vi "Dashboard Main.vi"() -> ()   [LabVIEW 2018]
uses:
  <vilib>/Utility/miscctls.llb/LVRowAndColumnTypeDef.ctl
  <vilib>/event_ctls.llb/eventvkey.ctl
  <vilib>/Rock Robotics/WPI/Dashboard/WPI_DashboardLogging Global.vi
  Personalities Tool/Main.vi
  <vilib>/Rock Robotics/Network Tables/NT Read Boolean.vi
  <vilib>/FTP/NI_FTP.lvlib
  Personalities Tool/Personalities Tool.lvlib
panel:
  in  "Camera Settings Right":T1={"Frame Rate"=30, "Compression"=30, "Size"=1, "DB Camera Config"=FALSE} {"Frame Rate" scale=1.0..30.0; "Compression" scale=100.0..-1.0; "Size" items=["640x480", "320x240", "160x120"]}
  in  "Camera Name Right":string(combo)="No Camera Selection"
  out "Camera Perf":string
  in  "Camera Settings":T1={"Frame Rate"=30, "Compression"=30, "Size"=1, "DB Camera Config"=FALSE} {"Frame Rate" scale=1.0..30.0; "Compression" scale=100.0..-1.0; "Size" items=["640x480", "320x240", "160x120"]}
  in  "TCP":refnum<k5>
  in  "Rec Mode":enum32{"Stop", "Record", "Playback"}(radio)
  out "Robot IP":string
  out "Image Message":string="Timeout in Camera Communications"
  in  "Dashboard Tab":T2(tab)
  out "Personality":string
  out "Elevator State":string
  out "Elevator Position":string
  in  "Select Auto":string(combo)="Select Autonomous ..."
  out "NT Connection":bool
  out "JS1 Z":dbl(slide) scale=-1.0..1.0 scale format="%#_2e"
  out "JS1 Graph":cluster{"X":dbl, "Y":dbl}[](graph)
  out "JS1 Buttons":T3
  out "JS2 Z":dbl(slide) scale=-1.0..1.0 scale format="%#_2e"
  out "JS2 Graph":cluster{"X":dbl, "Y":dbl}[](graph)
  out "JS2 Buttons":T3
  out "Mode":T4(ring)=enum."Auto Disabled"
  out "Right Camera Perf":cluster{"Bandwidth (Mbps)":dbl, "FPS":dbl}
  out "BirdBeak State":bool
  out "Camera Image Right":T5(plugin-control)
  in  "DB/String 9":string
  in  "DB/String 8":string
  in  "DB/String 7":string
  in  "DB/String 6":string
  in  "DB/String 5":string
  in  "DB/String 4":string
  in  "DB/String 3":string
  in  "DB/String 2":string
  in  "DB/String 1":string
  in  "DB/String 0":string
  in  "DB/Slider 0":dbl(slide) scale=0.0..5.0
  in  "DB/Slider 1":dbl(slide) scale=0.0..5.0
  in  "DB/Slider 2":dbl(slide) scale=0.0..5.0
  in  "DB/Slider 3":dbl(slide) scale=0.0..5.0
  out "DB/LED 3":bool
  out "DB/LED 2":bool
  out "DB/LED 1":bool
  out "DB/LED 0":bool
  in  "DB/Button 3":bool
  in  "DB/Button 2":bool
  in  "DB/Button 1":bool
  in  "DB/Button 0":bool caption="New Name"
  in  "Open Personalities Tool":bool
  in  "Retrieve File":bool
  in  "Click me if this is a new Driver Station":bool
  out "String":string
  out "Error":bool
  in  "Transfer File":bool
  in  "Edit File":bool
  in  "File":u16(ring) items=["CodeConstants.ini", "CodeConstants_Comp.ini", "CodeConstants_Prac.ini", "ConfigFileSettings.ini", "ElevatorBot.ini", "NewConfigFile.ini", "Outlaw.ini", "PacBot.ini"]
  in  "Test Slider":dbl(slide) scale=0.0..100.0 scale format="%#_3g"
  in  "On/Off":bool caption="Solenoid"
  in  "Test Name":u16(ring) items=["Select the test to run..."]
  in  "Test Tree":string(tree)
  in  "Motor":cluster{"Value":dbl, "Enable":bool} {"Value" scale=-1.0..1.0 scale format="%#_3g"}
  out "Progress":T6 {"Test Progress" scale=0.0..100.0}
  in  "Rev/Fwd":cluster{"Forward":bool, "Reverse":bool}
  in  "Test Ring":u16(ring) items=["Monochrome", "Color"]
  out "Cmd Status":string
  in  "Execute Command":bool
  in  "Command Params":string[][](table)
  in  "Command Selection":i32(listbox)
  in  "CheckList":i32(listbox)
  out "Tree":string(tree)
  out "Camera Image":T5(plugin-control)
  out "Background":bool
  in  "Camera Name":string(combo)="No Camera Selection"
  # "HW"
  # "HW"
  # "Joysticks"
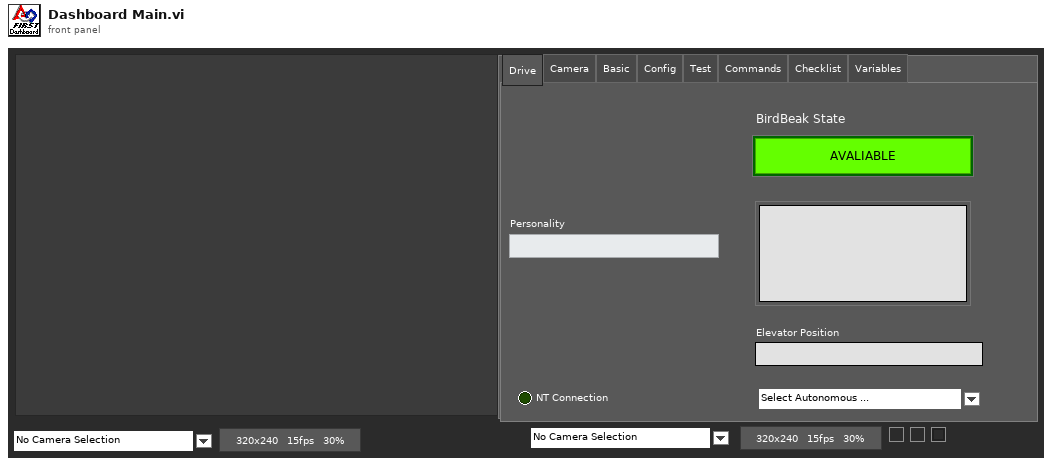
[diagram p1: front panel]
types:
  T1 = cluster{"Frame Rate":i32, "Compression":i32, "Size":u16, "DB Camera Config":bool}
  T2 = enum32{"Drive", "Camera", "Basic", "Config", "Test", "Commands", "Checklist", "Variables"}
  T3 = cluster{bool, bool, bool, bool, bool, bool, bool, bool, bool, bool, bool, bool}
  T4 = enum8{"Tele-Op Disabled", "Tele-Op Enabled", "Auto Disabled", "Auto Enabled", "Test Disabled", "Test Enabled", "Disconnected", "No Code", "E-Stop"}
  T5 = typedef "IMAQ Image.ctl" = refnum<image>
  T6 = cluster{"Test Progress":u8, "Test Progress Text":string}
  T7 = cluster{"Save Path":path, "Interval (s)":dbl, "Keep":i32}
  T8 = enum32{"Drive", "Camera", "Basic", "Custom", "Test", "Commands", "Checklist", "Variables"}
  T9 = typedef "Image Type" = u32
  T10 = cluster{"IDs":cluster{"RPC field ID":u16, "Unique ID":u16}, "String":string}
  T11 = cluster{"Error Strings":string, "Disable Counts":cluster{u16, u16}, "Rail Faults":cluster{u16, u16, u16}, "Robot IP":string, "DB Mode":u8, "Event Info":cluster{"Name":string, "Type":u8, "Number":u16, "Replay":u8}}
  T12 = cluster{"Storage":cluster{"Disk Free":u64, "RAM Block":u32, "RAM free":u32}, "CPU Utilization":cluster{"CPU % ISR":sgl, "CPU % Time Crit":sgl, "CPU % Timed Str":sgl, "CPU % High":sgl, "CPU % Above":sgl, "CPU % Normal":sgl, "CPU % Low":sgl}, "CAN":cluster{"% Bus Utilization":sgl, "Bus Off Cnt":u32, "TX_FIFO Full Cnt":u32, "Receive Error Cnt":u8, "Transmit Error Cnt":u8}, "HID":cluster{"HID Outputs":u32, "Rumble Low":u16, "Rumble High":u16}[]}
  T13 = cluster{"Status bits":cluster{"Test Mode":bool, "Autonomous":bool, "Enabled":bool, "Code Start":bool, "Brownout":bool, "Reserved 2":bool, "Reserved 3":bool, "E-Stop":bool}, "Code Trace":cluster{"Disabled":bool, "TeleOp":bool, "Auto":bool, "Test":bool}, "Controller Type":enum16{"unknown", "cRIO", "roboRio"}, "Code?":enum16{"unknown", "noCode", "code"}, "Battery V":dbl}
  T14 = cluster{"Control Bits":cluster{"TestMode":bool, "Autonomous":bool, "Enabled":bool, "FMS Present":bool, bool, bool, bool, "E-Stop":bool}, "Team Station ":u8, "Countdown":sgl, "Joystick Values":cluster{"Axes":dbl[], "Buttons":bool[], "POVs":i16[]}[]}
  T15 = cluster{"Axes":dbl[], "Buttons":bool[], "POVs":i16[]}[]
  T16 = cluster{"Axes":dbl[], "Buttons":bool[], "POVs":i16[]}
  T17 = cluster{"Buttons[0]":bool, "Buttons[1]":bool, "Buttons[2]":bool, "Buttons[3]":bool, "Buttons[4]":bool, "Buttons[5]":bool, "Buttons[6]":bool, "Buttons[7]":bool, "Buttons[8]":bool, "Buttons[9]":bool, "Buttons[10]":bool, "Buttons[11]":bool}
  T18 = cluster{"Camera Image":refnum<vi>, "Dashboard Tab":refnum<vi>, "Background":refnum<vi>, "Rec Mode":refnum<vi>, "Test Slider":refnum<vi>, "On/Off ":refnum<vi>, "Test Ring":refnum<vi>, "Rev/Fwd":refnum<vi>, "Test Name":refnum<vi>, "Motor":refnum<vi>, "Progress":refnum<vi>, "CheckList":refnum<vi>, "Tree":refnum<vi>, "Test Tree":refnum<vi>, "Command Params":refnum<vi>, "Command Selection":refnum<vi>, "Execute Command":refnum<vi>, "Cmd Status":refnum<vi>, "Camera Settings":refnum<vi>, "Camera Name":refnum<vi>, "Camera Perf":refnum<vi>, "Camera Settings Right":refnum<vi>, "Camera Name Right":refnum<vi>, "Camera Image Right":refnum<vi>}
  T19 = cluster{"Global Rectangle":i32[], "Contours":cluster{"Contour Type":u32, "ROI Type":u32, "Points":i32[]}[]}
  T20 = cluster{"Camera Name":string, string, "Saved DB Images Info":cluster{"Save Path":path, "Interval (s)":dbl, "Keep":i32}}
  T21 = cluster{"Camera Name Right":string, string, "Saved DB Images Info":cluster{"Save Path":path, "Interval (s)":dbl, "Keep":i32}}
  T22 = cluster{"Operation":enum16{"Update", "Clear"}, "Color Box":u32}[]
  T23 = enum32{"Invalid", "Standard", "Closed", "Hidden", "Minimized", "Maximized"}
  T24 = typedef "eventvkey.ctl" = enum16{"ASCII", "Enter", "Return", "Shift", "Ctrl", "Alt", "Cmd", "Opt", "Caps", "NumLock", "Clear", "Break", "Up", "Down", "Left", "Right", "Insert", "Delete", "Home", "End", "PageUp", "PageDown", "Escape", "Help", "Pause", "ScrollLock", "F1", "F2", "F3", "F4", "F5", "F6", "F7", "F8", "F9", "F10", "F11", "F12", "F13", "F14", "F15", "F16", "F17", "F18", "F19", "F20", "F21", "F22", "F23", "F24", "Play", "VolumeUp", "VolumeDown", "Mute", "Two Byte Char"}
  T25 = cluster{"Image Size":bool, "Image Type":bool, "Pixel Value":bool, "ROI Information":bool, "Zoom Factor":bool}
  T26 = cluster{"Operation":enum16{"Update", "Clear"}, "Color Box":u32}
  T27 = typedef "LVRowAndColumnTypeDef.ctl" = cluster{"Row":i32, "Column":i32}
  T28 = cluster{"Shift":bool, "Ctrl":bool, "Alt":bool, "Cmd":bool, "Opt":bool}
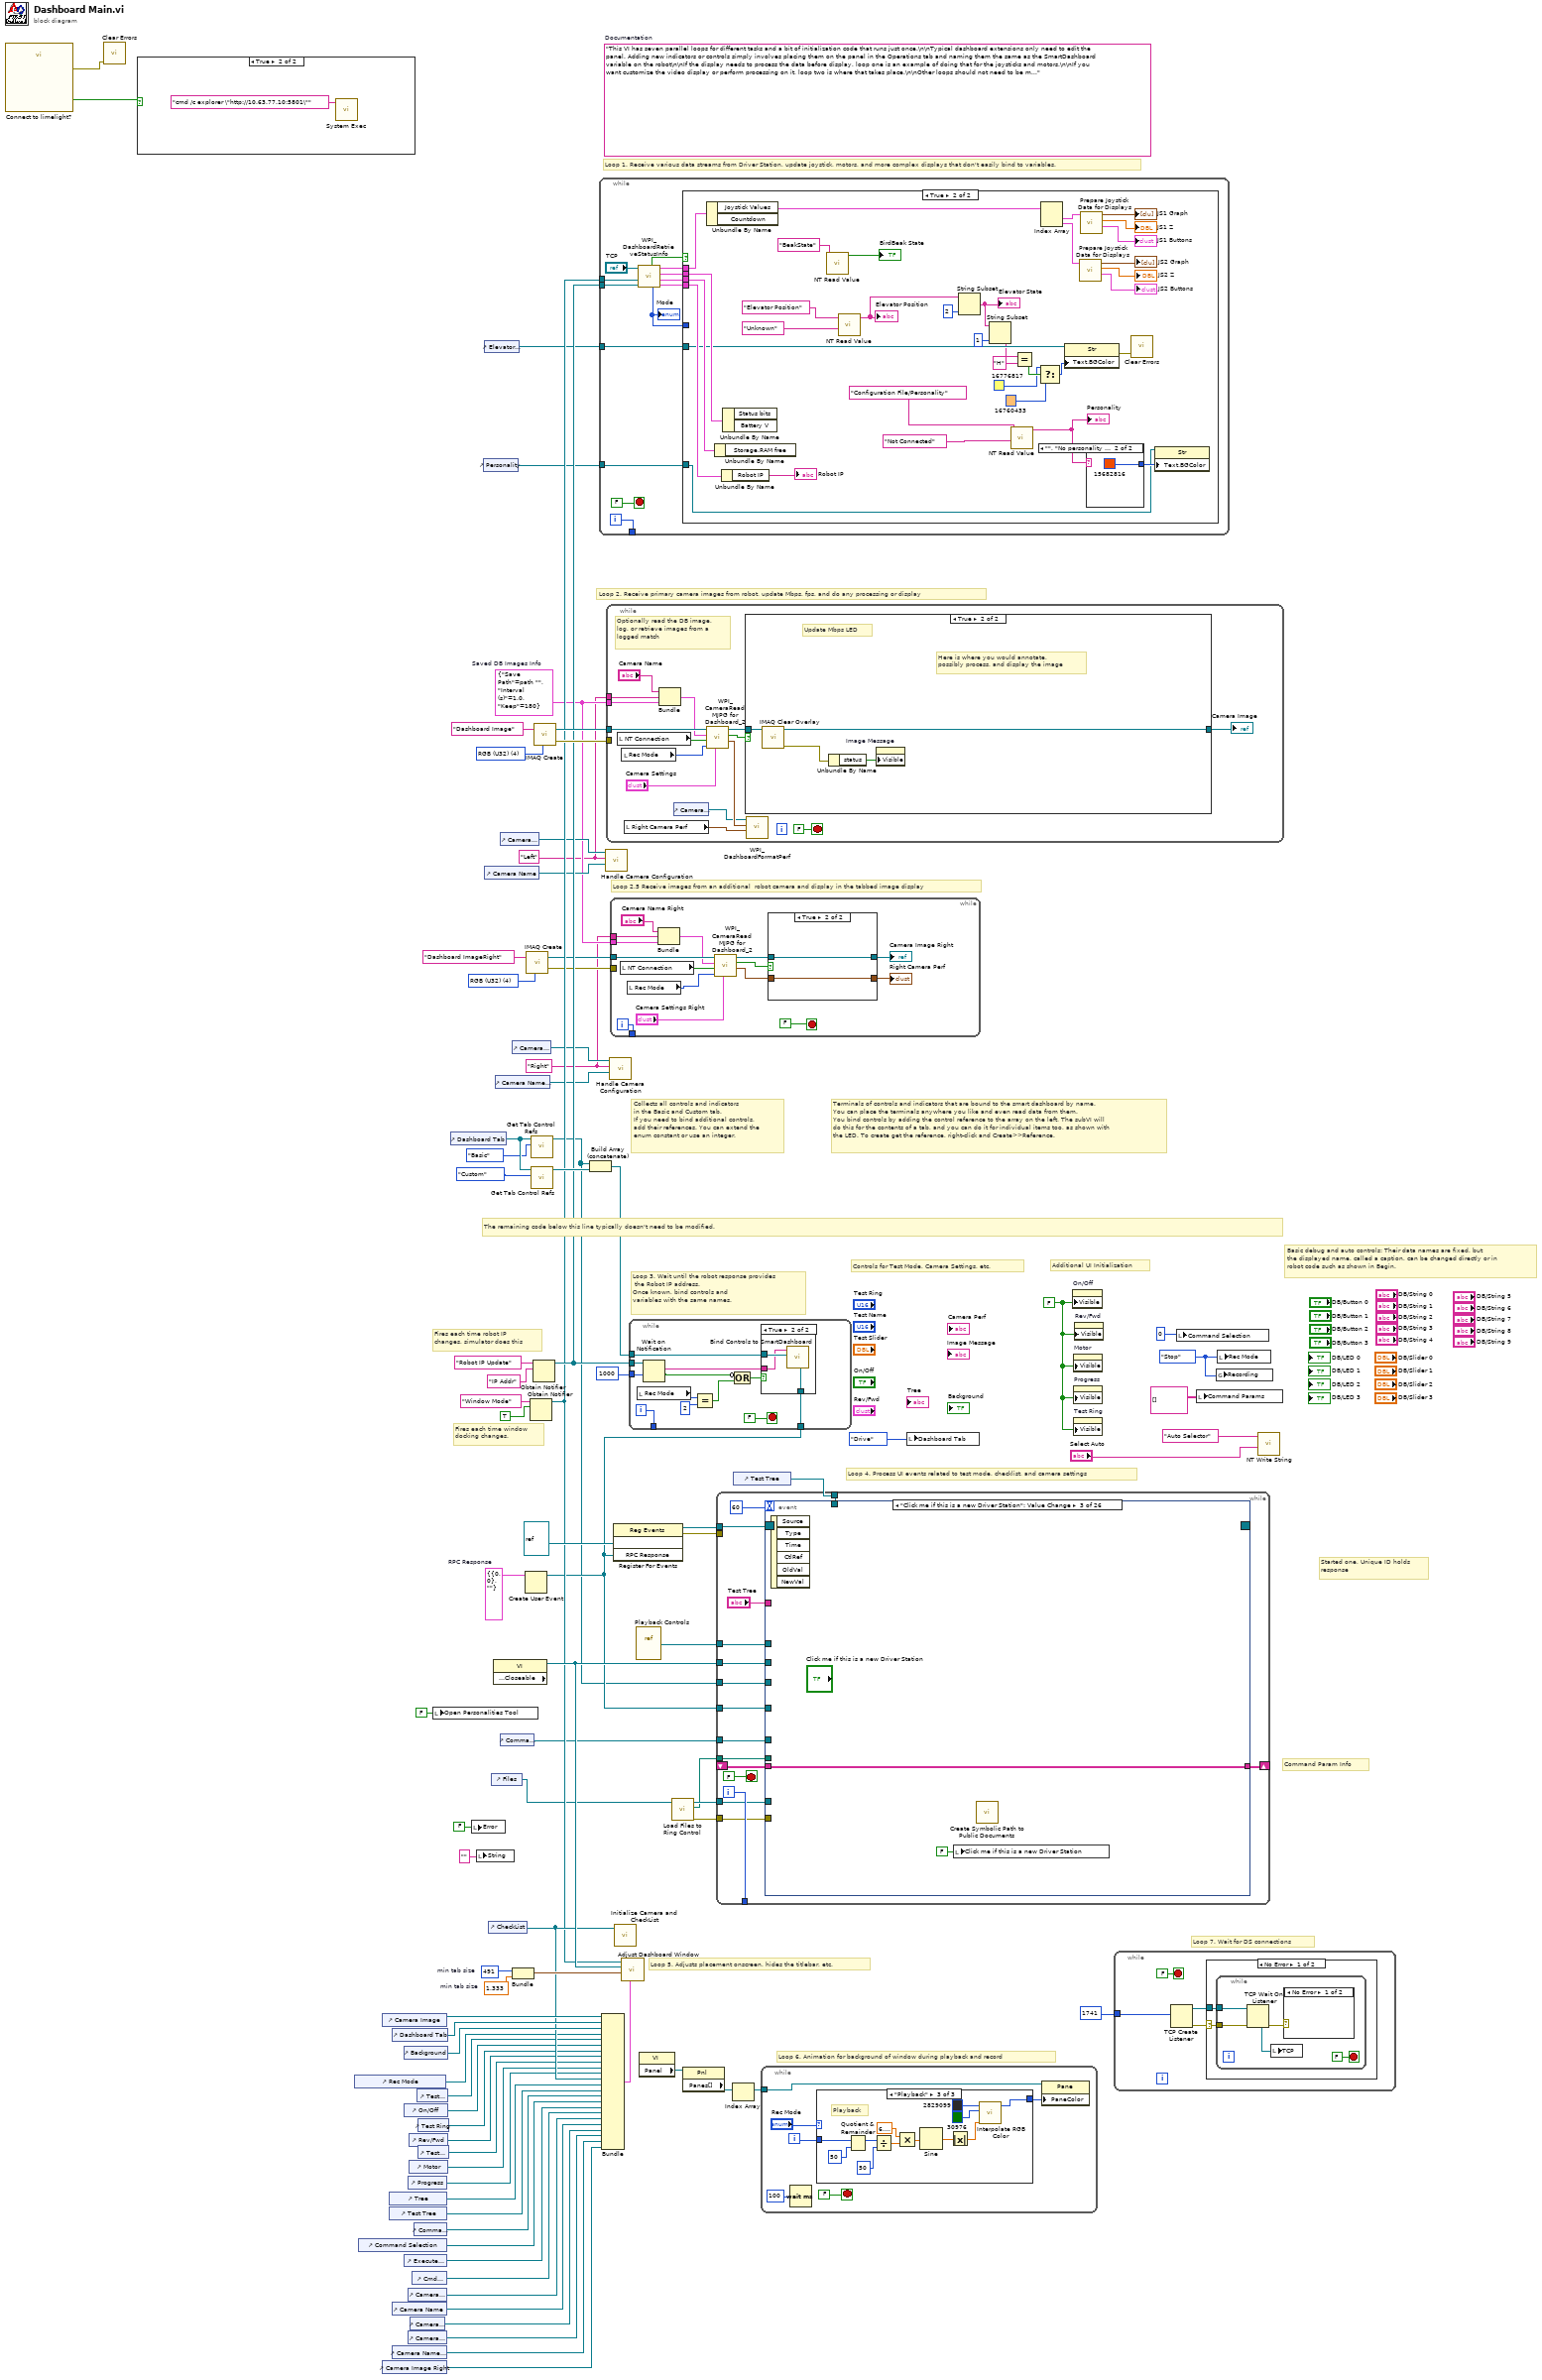
[diagram p0: block diagram]
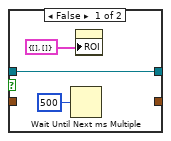
[diagram p3: hidden frame]
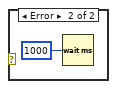
[diagram p4: hidden frame]
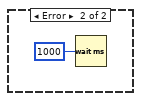
[diagram p5: hidden frame]
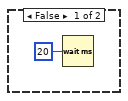
[diagram p6: hidden frame]
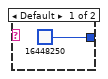
[diagram p7: hidden frame]
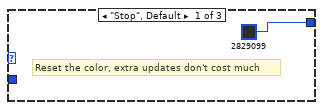
[diagram p8: hidden frame]
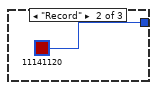
[diagram p9: hidden frame]
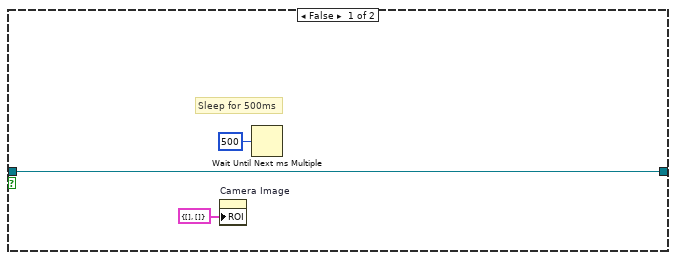
[diagram p11: hidden frame]
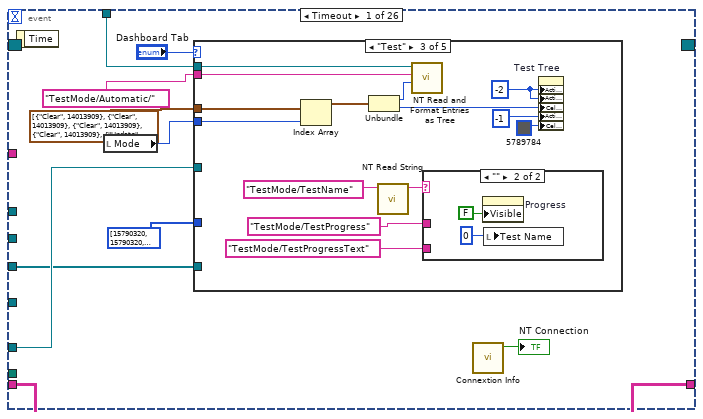
[diagram p12: hidden frame]
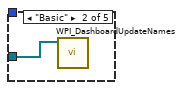
[diagram p14: hidden frame]
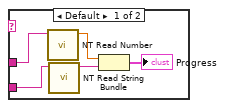
[diagram p15: hidden frame]
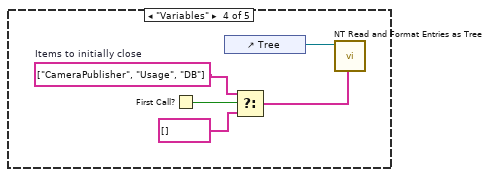
[diagram p16: hidden frame]
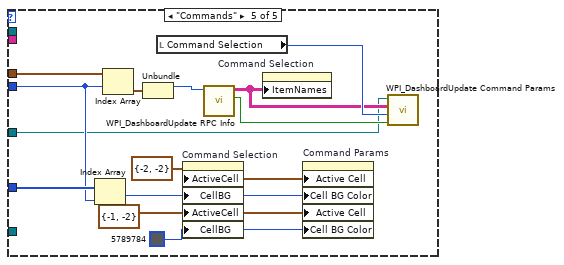
[diagram p17: hidden frame]
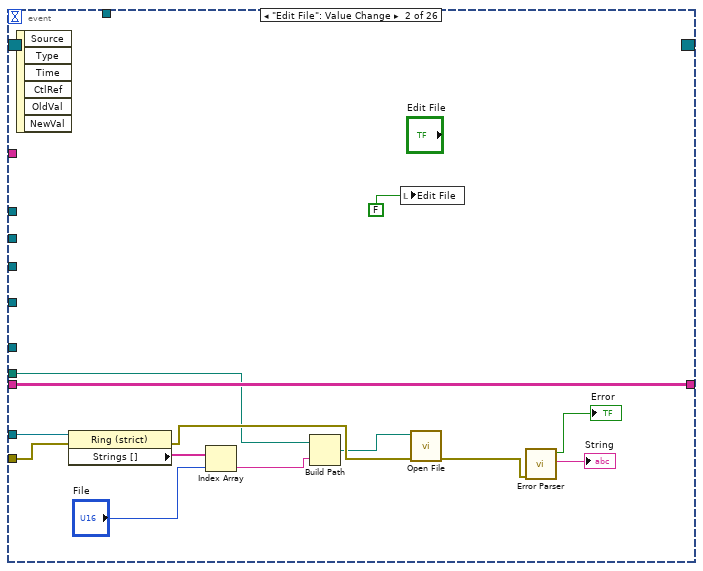
[diagram p18: hidden frame]
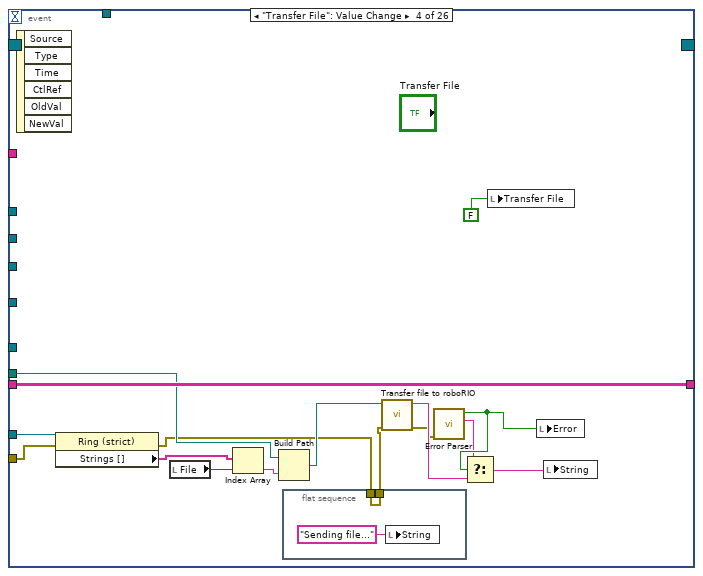
[diagram p19: hidden frame]
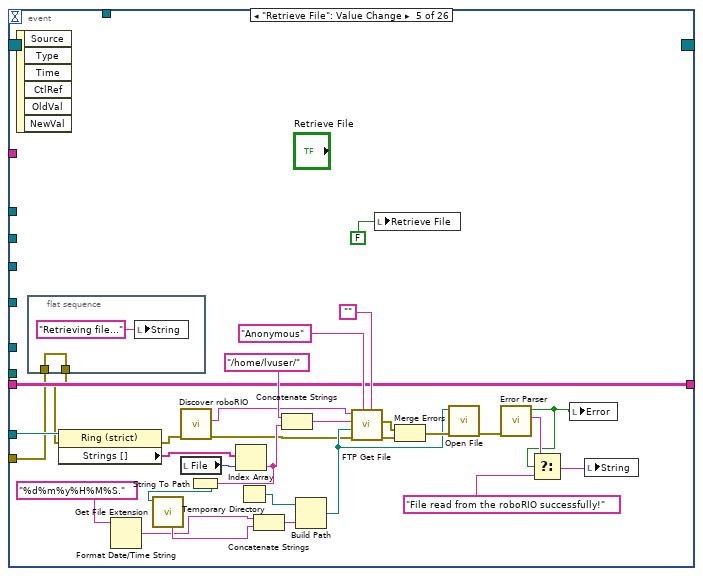
[diagram p20: hidden frame]
diagram:
  w14 = T7 {"Save Path"=path "", "Interval (s)"=1.0, "Keep"=180}  # Saved DB Images Info
  w13 = "Right"
  w12 = "Left"
  w24 = T9 4 items=["Grayscale (U8)", "Grayscale (I16)", "Grayscale (SGL)", "Complex (CSG)", "RGB (U32)", "HSL (U32)", "RGB (U64)"] ("Image Type")
  w40 = T10 {"IDs"={"RPC field ID"=0, "Unique ID"=0}, "String"=""}  # RPC Response
  w63 = 491  # min tab size
  w62 = 1.333  # min tab size
  w70 = enum32{"Stop", "Record", "Playback"}."Stop" ("Rec Mode")
  w47 = FALSE ("Visible")
  (unwired) "This VI has seven parallel loops for different tasks and a bit of initialization code that runs just once.\n\nTypical dashboard extensions only need to edit the panel. Adding new indicators or controls simply involves placing them on the panel in the Operations tab and naming them the same as the SmartDashboard variable on the robot\n\nIf the display needs to process the data before display, loop one is an example of doing that for the joysticks and motors.\n\nIf you want customize the video display or perform processing on it, loop two is where that takes place.\n\nOther loops should not need to be modified. They are pretty standard, and document the task they perform."  # Documentation
  w87 = T9 4 items=["Grayscale (U8)", "Grayscale (I16)", "Grayscale (SGL)", "Complex (CSG)", "RGB (U32)", "HSL (U32)", "RGB (U64)"] ("Image Type")
  # "Loop 2.5 Receive images from an additional  robot camera and display in the tabbed image display"
  # "Command Param Info"
  # "Started one, Unique ID holds\nresponse"
  # "Loop 7. Wait for DS connections"
  # "Basic debug and auto controls: Their data names are fixed, but\nthe displayed name, called a caption, can be changed directly or in\nrobot code such as shown in Begin."
  # "Controls for Test Mode, Camera Settings, etc."
  # "Additional UI Initialization"
  # "Loop 6. Animation for background of window during playback and record"
  # "Fires each time robot IP\nchanges, simulator does this"
  # "Fires each time window\ndocking changes."
  # "Collects all controls and indicators\nin the Basic and Custom tab.\nIf you need to bind additional controls,\nadd their references. You can extend the\nenum constant or use an integer."
  # "The remaining code below this line typically doesn't need to be modified."
  # "Loop 4. Process UI events related to test mode, checklist, and camera settings"
  # "Terminals of controls and indicators that are bound to the smart dashboard by name.\nYou can place the terminals anywhere you like and even read data from them.\nYou bind controls by adding the control reference to the array on the left. The subVI will\ndo this for the contents of a tab, and you can do it for individual items too, as shown with\nthe LED. To create get the reference, right-click and Create>>Reference."
  # "Loop 3. Wait until the robot response provides\n the Robot IP address.\nOnce known, bind controls and\nvariables with the same names."
  # "Loop 5. Adjusts placement onscreen, hides the titlebar, etc."
  # "Loop 1. Receive various data streams from Driver Station, update joystick, motors, and more complex displays that don't easily bind to variables."
  # "Loop 2. Receive primary camera images from robot, update Mbps, fps, and do any processing or display"
  n1 = call "Connect to limelight?"() -> ("Yes"=w5:bool, "error out"=w4:errorcluster)  [unwired: 18 in]
  n2 = call <vilib>:"Clear Errors.vi"("error in (no error)"=w4) -> ()  [unwired: 5 in, 2 out]
  n3 = case shown="True" w5 {
    frame False {
    }
    frame True {
      n4 = call <vilib>:"System Exec.vi"("command line"="cmd /c explorer \"http://10.63.77.10:5801\"") -> ()  [unwired: 7 in, 4 out]
    }
  }
  n5 = control-ref of="Rec Mode"() -> (w53:refnum<vi>)
  n6 = control-ref of="Command Selection"() -> (w39:refnum<vi>)
  n7 = control-ref of="Camera Image Right"() -> (w17:refnum<vi>)
  n8 = control-ref of="Camera Image"() -> (w65:refnum<vi>)
  n9 = control-ref of="Tree"() -> (w57:refnum<vi>)
  n10 = control-ref of="Test Tree"() -> (w56:refnum<vi>)
  n11 = control-ref of="Dashboard Tab"() -> (w64:refnum<vi>)
  n12 = control-ref of="Camera Name"() -> (w30:refnum<vi>)
  n13 = control-ref of="Camera Name Right"() -> (w18:refnum<vi>)
  n14 = control-ref of="Execute Command"() -> (w41:refnum<vi>)
  n15 = control-ref of="Background"() -> (w60:refnum<vi>)
  n16 = control-ref of="On/Off"() -> (w51:refnum<vi>)
  n17 = control-ref of="Progress"() -> (w48:refnum<vi>)
  n18 = control-ref of="Camera Settings"() -> (w31:refnum<vi>)
  n19 = control-ref of="Camera Settings Right"() -> (w19:refnum<vi>)
  n20 = control-ref of="Rev/Fwd"() -> (w49:refnum<vi>)
  n21 = control-ref of="Motor"() -> (w54:refnum<vi>)
  n22 = control-ref of="Camera Perf"() -> (w29:refnum<vi>)
  n23 = control-ref of="Cmd Status"() -> (w35:refnum<vi>)
  n24 = control-ref of="Command Params"() -> (w42:refnum<vi>)
  n25 = control-ref of="Test Slider"() -> (w52:refnum<vi>)
  n26 = control-ref of="Test Ring"() -> (w50:refnum<vi>)
  n27 = control-ref of="Test Name"() -> (w55:refnum<vi>)
  n28 = local write "Open Personalities Tool"(FALSE ("Open Personalities Tool")) -> ()
  n29 = control-ref of="Dashboard Tab"() -> (w68:refnum<vi>)
  n30 = local write "Error"(FALSE ("Error")) -> ()
  n31 = local write "String"("" ("String")) -> ()
  n32 = control-ref of="Personality"() -> (w2:refnum<vi>)
  n33 = control-ref of="Elevator State"() -> (w3:refnum<vi>)
  n34 = control-ref of="Camera Name"() -> (w32:refnum<vi>)
  n35 = control-ref of="CheckList"() -> (w58:refnum<vi>)
  n36 = control-ref of="Files"() -> (w11:refnum<vi>)
  n37 = property class="VI" props=["Front Panel.Closeable"]() -> (reference out=w69:refnum<vi>)  [unwired: 2 in, 2 out]
  n38 = control-ref of="Camera Name Right"() -> (w20:refnum<vi>)
  n39 = control-ref of="Camera Settings"() -> (w33:refnum<vi>)
  n40 = control-ref of="Command Params"() -> (w34:refnum<vi>)
  n41 = control-ref of="Camera Settings Right"() -> (w21:refnum<vi>)
  n42 = Bundle("min tab size"=w63, "min tab size"=w62) -> (w61:cluster{"min tab size":i32, "min tab size":dbl})  [unwired: 1 in]
  n43 = Create User Event(user event datatype=w40) -> (user event=w36:refnum<user-event>)  [unwired: 1 in, 1 out]
  n44 = call "IMAQ Create"("Image Name"="Dashboard ImageRight", "Image Type"=w24) -> ("New Image"=w23:T5, "error out"=w22:errorcluster)  [unwired: 2 in, 1 out]
  n45 = Obtain Notifier(name (unnamed)="Window Mode", notification data type=TRUE) -> (notifier out=w45:refnum<notifier>)  [unwired: 2 in, 2 out]
  n46 = call <vilib>:"Get Tab Control Refs.vi"("Page Index"=T8."Basic" ("Dashboard Tab"), "TabControl in"=w68) -> ("ControlsOnPage"=w28:refnum<vi>[])  [unwired: 9 in]
  n47 = call <vilib>:"Get Tab Control Refs.vi"("Page Index"=T8."Custom" ("Dashboard Tab"), "TabControl in"=w68) -> ("ControlsOnPage"=w67:refnum<vi>[])  [unwired: 9 in]
  n48 = Obtain Notifier(name (unnamed)="Robot IP Update", notification data type="IP Addr" ("name (unnamed)")) -> (notifier out=w46:refnum<notifier>)  [unwired: 2 in, 2 out]
  n49 = call "IMAQ Create"("Image Name"="Dashboard Image", "Image Type"=w87) -> ("New Image"=w85:T5, "error out"=w84:errorcluster)  [unwired: 2 in, 1 out]
  n50 = Build Array (concatenate)(w28, w67) -> (w66:refnum<vi>[])
  n51 = while {
    tunnel: [w100] -> _
    tunnel: w46 -> [w94]
    tunnel: w45 -> [w91]
    tunnel: w3 -> [w90]
    tunnel: w2 -> [w89]
    i -> [w100]
    stop <- FALSE stop-if-true
    n52 = call <vilib>:"WPI_DashboardRetrieveStatusInfo.vi"("Binding Refnum"=w94, "Window Mode Notifier"=w91, "TCP Cnx"="TCP") -> ("Power and Errors"=w95:T11, "Robot Metrics"=w98:T12, "Status Info"=w99:T13, "Control Info"=w96:T14, "Robot Mode"=w93:T4, "Process?"=w97:bool)  [unwired: 3 in]
    "Mode" <- w93
    n53 = case shown="True" w97 {
      tunnel: w99 -> [_ w137]
      tunnel: w98 -> [_ w136]
      tunnel: w96 -> [_ w135]
      tunnel: w95 -> [_ w134]
      tunnel: w93 -> [_ _]
      tunnel: w90 -> [_ w117]
      tunnel: w89 -> [_ w103]
      frame False {
        n54 = Wait (ms)(milliseconds to wait=u32 20) -> ()  [unwired: 1 out]
      }
      frame True {
        n55 = Unbundle By Name(w135) -> ("Joystick Values"=w133:T15)  [unwired: 1 out]
        n56 = Unbundle By Name(w136) -> ()  [unwired: 1 out]
        n57 = Unbundle By Name(w134) -> ("Robot IP"=→"Robot IP":string)
        n58 = Unbundle By Name(w137) -> ()  [unwired: 2 out]
        n59 = call-poly <vilib>:"NT Read Value.vi"("Name"="BeakState") -> ("Boolean"=→"BirdBeak State":bool)  [unwired: 9 in, 1 out]
        n60 = call-poly <vilib>:"NT Read Value.vi"("Default Value"="Unknown", "Name"="Elevator Position") -> ("String"=w119:string)  [unwired: 8 in, 1 out]
        "Elevator Position" <- w119
        n61 = String Subset(string=w119, length (rest)=2 ("length (rest)")) -> (substring=w116:string)  [unwired: 1 in]
        "Elevator State" <- w116
        n62 = String Subset(string=w116, length (rest)=1 ("length (rest)")) -> (substring=w114:string)  [unwired: 1 in]
        n63 = call-poly <vilib>:"NT Read Value.vi"("Default Value"="Not Connected", "Name"="Configuration File/Personality") -> ("String"=w104:string)  [unwired: 8 in, 1 out]
        "Personality" <- w104
        n64 = Equal?(x=w114, y="H") -> (x = y?=w111:bool)
        n65 = Select(t=u32 16776817, s=w111, f=u32 16760433) -> (s? t:f=w112:u32)
        n66 = Index Array(array=w133) -> (element #1=w132:T16, element #2=w128:T16)  [unwired: 2 in]
        n67 = property class="Str"(reference=w117, "Text.BGColor"=w112) -> (error out=w108:errorcluster)  [unwired: 1 in, 1 out]
        n68 = call "Prepare Joystick Data for Displays.vi"("Joystick Values"=w128) -> ("Buttons"=→"JS2 Buttons":T17, "Z Axis"=→"JS2 Z":dbl, "Cartesian Data"=→"JS2 Graph":cluster{"X axis":dbl, "X axis":dbl}[])  [unwired: 8 in]
        n69 = call "Prepare Joystick Data for Displays.vi"("Joystick Values"=w132) -> ("Buttons"=→"JS1 Buttons":T17, "Z Axis"=→"JS1 Z":dbl, "Cartesian Data"=→"JS1 Graph":cluster{"X axis":dbl, "X axis":dbl}[])  [unwired: 8 in]
        n70 = case shown="\"\", \"No personality found.\", \"Not Connected\"" w104 {
          tunnel: [u32 16448250 u32 15682816] -> w105
          frame Default {
          }
          frame "", "No personality found.", "Not Connected" {
          }
        }
        n71 = call <vilib>:"Clear Errors.vi"("error in (no error)"=w108) -> ()  [unwired: 5 in, 2 out]
        n72 = property class="Str"(reference=w103, "Text.BGColor"=w105) -> ()  [unwired: 1 in, 2 out]
      }
    }
  }
  n73 = Bundle("Camera Image"=w65, "Dashboard Tab"=w64, "Background"=w60, "Rec Mode"=w53, "Test Slider"=w52, "On/Off"=w51, "Test Ring"=w50, "Rev/Fwd"=w49, "Test Name"=w55, "Motor"=w54, "Progress"=w48, "CheckList"=w58, "Tree"=w57, "Test Tree"=w56, "Command Params"=w42, "Command Selection"=w39, "Execute Command"=w41, "Cmd Status"=w35, "Camera Settings"=w31, "Camera Name"=w30, "Camera Perf"=w29, "Camera Settings Right"=w19, "Camera Name Right"=w18, "Camera Image Right"=w17) -> (w59:T18)  [unwired: 1 in]
  n74 = call "Handle Camera Configuration.vi"("CameraNameRef"=w32, "Display Name"=w12, "ClusterRef"=w33) -> ()  [unwired: 9 in]
  n75 = while {
    tunnel: w85 -> [w153]
    tunnel: w84 -> [_]
    tunnel: w14 -> [w146]
    tunnel: w12 -> [w143]
    stop <- FALSE stop-if-true
    # "Optionally read the DB image,\nlog, or retrieve images from a\nlogged match"
    n76 = local read "NT Connection"() -> (w147:bool)
    n77 = local read "Rec Mode"() -> (w150:enum32{"Stop", "Record", "Playback"})
    n78 = local read "Right Camera Perf"() -> (w141:cluster{"Bandwidth (Mbps)":dbl, "FPS":dbl})
    n79 = Bundle("Camera Name"="Camera Name", w143, "Saved DB Images Info"=w146) -> (w145:T20)  [unwired: 1 in]
    n80 = control-ref of="Camera Perf"() -> (w140:refnum<vi>)
    n81 = call <vilib>:"WPI_CameraRead MJPG for Dashboard_2.vi"("Camera Settings"="Camera Settings", "Rec Mode"=w150, "NT Connection"=w147, "Capture Info"=w145, "Image in"=w153) -> ("perf info"=w142:cluster{"Bandwidth (Mbps)":dbl, "fps":dbl}, "Active"=w151:bool, "Image\\ out"=w152:T5)  [unwired: 4 in]
    n82 = case shown="True" w151 {
      tunnel: w152 -> [w156 w159]
      tunnel: [w156 w158] -> w148
      frame False {
        # "Sleep for 500ms"
        n83 = property on="Camera Image" class="ImageControl"("ROI"=T19 {"Global Rectangle"=[], "Contours"=[]}) -> ()  [unwired: 2 in, 2 out]
        n84 = Wait Until Next ms Multiple(millisecond multiple=u32 500) -> ()  [unwired: 1 out]
      }
      frame True {
        # "Here is where you would annotate,\npossibly process, and display the image"
        # "Update Mbps LED"
        n85 = call "IMAQ Clear Overlay"("Image"=w159) -> ("error out"=w160:errorcluster, "Image Out"=w158:T5)  [unwired: 2 in, 7 out]
        n86 = Unbundle By Name(w160) -> ("status"=w161:bool)
        n87 = property on="Image Message" class="Str"("Visible"=w161) -> ()  [unwired: 2 in, 2 out]
      }
    }
    "Camera Image" <- w148
    n88 = call <vilib>:"WPI_DashboardFormatPerf.vi"("Right Camera Perf"=w141, "Performance"=w142, "String in"=w140) -> ()  [unwired: 9 in]
  }
  n89 = call "Handle Camera Configuration.vi"("CameraNameRef"=w20, "Display Name"=w13, "ClusterRef"=w21) -> ()  [unwired: 9 in]
  n90 = while {
    tunnel: w23 -> [w176]
    tunnel: w22 -> [_]
    tunnel: [w171] -> _
    tunnel: w14 -> [w167]
    tunnel: w13 -> [w164]
    i -> [w171]
    stop <- FALSE stop-if-true
    n91 = local read "NT Connection"() -> (w168:bool)
    n92 = local read "Rec Mode"() -> (w175:enum32{"Stop", "Record", "Playback"})
    n93 = Bundle("Camera Name Right"="Camera Name Right", w164, "Saved DB Images Info"=w167) -> (w166:T21)  [unwired: 1 in]
    n94 = call <vilib>:"WPI_CameraRead MJPG for Dashboard_2.vi"("Camera Settings"="Camera Settings Right", "Rec Mode"=w175, "NT Connection"=w168, "Capture Info"=w166, "Image in"=w176) -> ("perf info"=w162:cluster{"Bandwidth (Mbps)":dbl, "fps":dbl}, "Active"=w170:bool, "Image\\ out"=w173:T5)  [unwired: 4 in]
    n95 = case shown="True" w170 {
      tunnel: w173 -> [w178 w181]
      tunnel: [w178 w181] -> w169
      tunnel: [_ w180] -> w163
      tunnel: w162 -> [_ w180]
      frame False {
        n96 = Wait Until Next ms Multiple(millisecond multiple=u32 500) -> ()  [unwired: 1 out]
        n97 = property on="Camera Image Right" class="ImageControl"("ROI"=T19 {"Global Rectangle"=[], "Contours"=[]}) -> ()  [unwired: 2 in, 2 out]
      }
      frame True {
      }
    }
    "Camera Image Right" <- w169
    "Right Camera Perf" <- w163
  }
  n98 = register-events(refnum<vi> refnum, w36) -> (reference out=w74:refnum<event-registration>, error out=w73:errorcluster)  [unwired: 2 in]
  n99 = call "Initialize Camera and CheckList.vi"("ListBox in"=w58) -> ()  [unwired: 11 in]
  n100 = call "Adjust Dashboard Window.vi"("Sizing Refnums"=w59, "Size Constraints"=w61, "VI"=w69, "WIn Mode"=w45) -> ()  [unwired: 8 in]
  n101 = while {
    tunnel: w66 -> [w193]
    tunnel: w46 -> [w191]
    tunnel: [w189] -> _
    tunnel: u32 1000 ("milliseconds to wait") -> [w188]
    tunnel: w36 -> [w182]
    i -> [w189]
    stop <- FALSE stop-if-true
    n102 = local read "Rec Mode"() -> (w184:enum32{"Stop", "Record", "Playback"})
    n103 = Wait on Notification(notifier=w191, timeout in ms (-1)=w188) -> (notification=w190:string, timed out?=w186:bool)  [unwired: 2 in, 2 out]
    n104 = Equal?(x=w184, y=u16 2 ("Rec Mode")) -> (x = y?=w185:bool)
    n105 = Compound Arithmetic op=OR(invert w186, w185) -> (w187:bool)
    n106 = case shown="True" w187 {
      tunnel: w193 -> [_ w196]
      tunnel: w190 -> [_ w195]
      tunnel: w182 -> [_ w194]
      frame False {
      }
      frame True {
        n107 = call <vilib>:"Bind Controls to SmartDashboard.vi"("RPC ref"=w194, "Bound Control Refs"=w196, "Server IP Address"=w195) -> ()  [unwired: 9 in]
      }
    }
  }
  n108 = vi-ref "Playback Controls.vi"() -> (w75:refnum<vi>)
  n109 = property class="VI"() -> ("Panel"=w77:refnum<vi>)  [unwired: 2 in, 2 out]
  n110 = call "Load Files to Ring Control.vi"("Ring in"=w11) -> ("error out"=w9:errorcluster, "Path to files"=w8:path, "Ring out"=w10:refnum<vi>)  [unwired: 8 in]
  n111 = property class="Pnl"(reference=w77) -> ("Panes[]"=w78:refnum<vi>[])  [unwired: 1 in, 2 out]
  n112 = Index Array(array=w78) -> (element=w76:refnum<vi>)  [unwired: 1 in]
  n113 = control-ref of="Test Tree"() -> (w79:refnum<vi>)
  n114 = while {
    tunnel: [w209] -> _
    tunnel: w79 -> [w208]
    tunnel: w75 -> [w207]
    tunnel: w74 -> [w206]
    tunnel: w73 -> [_]
    tunnel: w69 -> [w205]
    tunnel: w36 -> [w204]
    tunnel: w34 -> [w203]
    shift-right: [w202] -> _
    shift-left: _ -> [w201]
    tunnel: w28 -> [w200]
    tunnel: w10 -> [w199]
    tunnel: w9 -> [w198]
    tunnel: w8 -> [w197]
    i -> [w209]
    stop <- FALSE stop-if-true
    n115 = event shown="[2] \"Click me if this is a new Driver Station\": Value Change" {
      selector: w206 -> [_ _ _ _ _ _ _ _ _ _ _ _ _ _ _ _ _ _ _ _ _ _ _ _ _ _]
      dyn-events: [_ _ _ _ _ _ _ _ _ _ _ _ _ _ _ _ _ _ _ _ _ w560 _ _ _ _] -> _
      timeout: u32 60 ("milliseconds to wait") -> [_ _ _ _ _ _ _ _ _ _ _ _ _ _ _ _ _ _ _ _ _ _ _ _ _ _]
      tunnel: w208 -> [w221 _ _ _ _ _ _ _ _ _ _ _ _ _ _ _ _ _ _ _ _ _ _ _ _ _]
      tunnel: "Test Tree" -> [_ _ _ _ _ _ _ _ _ _ _ _ _ _ _ _ w527 w535 w537 w541 w549 _ _ _ _ _]
      tunnel: w207 -> [_ _ _ _ _ _ _ _ _ _ _ _ _ _ _ _ _ _ _ _ _ w562 _ w580 _ _]
      tunnel: w205 -> [_ _ _ _ _ _ _ _ _ _ _ _ _ _ _ _ _ _ _ _ _ w558 _ _ _ _]
      tunnel: w204 -> [_ _ _ _ _ _ _ _ _ _ _ _ _ _ _ _ _ _ _ _ _ w556 _ _ _ _]
      tunnel: w203 -> [w216 _ _ _ _ _ _ _ _ _ _ w478 _ _ _ _ _ _ _ _ _ _ _ _ _ _]
      tunnel: [w215 w275 w277 w293 w314 w336 w355 w457 w462 w471 w475 w476 w485 w495 w502 w514 w526 w533 w536 w540 w548 w555 w575 w577 w581 w594] -> w202
      tunnel: w201 -> [w215 w275 w277 w293 w314 w336 w355 w457 w462 w471 w475 w476 _ _ w502 w514 w526 w533 w536 w540 w548 w555 w575 w577 w581 w594]
      tunnel: w200 -> [w213 _ _ _ _ _ _ _ _ _ _ _ _ _ _ _ _ _ _ _ _ _ _ _ _ _]
      tunnel: w199 -> [_ w274 _ w291 w313 _ _ _ _ _ _ _ _ _ _ _ _ _ _ _ _ _ _ _ _ _]
      tunnel: w198 -> [_ w273 _ w281 w299 _ _ _ _ _ _ _ _ _ _ _ _ _ _ _ _ _ _ _ _ _]
      tunnel: w197 -> [_ w263 _ w288 _ _ _ _ _ _ _ _ _ _ _ _ _ _ _ _ _ _ _ _ _ _]
      event Timeout {
        n116 = event-data() -> ()  [unwired: 1 in, 1 out]
        n117 = local read "Mode"() -> (w218:T4)
        n118 = case shown="\"Test\"" "Dashboard Tab" {
          tunnel: w221 -> [_ _ w237 _ _]
          tunnel: "TestMode/Automatic/" ("Name Pattern") -> [_ _ w236 _ _]
          tunnel: T22 [{"Operation"=enum."Clear", "Color Box"=14013909}, {"Operation"=enum."Clear", "Color Box"=14013909}, {"Operation"=enum."Clear", "Color Box"=14013909}, {"Operation"=enum."Clear", "Color Box"=14013909}, {"Operation"=enum."Update", "Color Box"=14013909}, {"Operation"=enum."Update", "Color Box"=16777215}, {"Operation"=enum."Clear", "Color Box"=14013909}, {"Operation"=enum."Clear", "Color Box"=14013909}, {"Operation"=enum."Clear", "Color Box"=14013909}] -> [_ _ w229 _ w257]
          tunnel: w218 -> [_ _ w228 _ w256]
          tunnel: u32[] [15790320, 15790320, 15790320, 15790320, 16777215, 16777215, 15790320, 15790320, 15790320] -> [_ _ _ _ w262]
          tunnel: w216 -> [_ _ _ _ w250]
          tunnel: w213 -> [_ w223 _ _ _]
          frame "Config", Default {
          }
          frame "Basic" {
            n119 = call <vilib>:"WPI_DashboardUpdateNames.vi"("Controls on Tab"=w223) -> ()  [unwired: 11 in]
          }
          frame "Test" {
            w235 = -2 ("Active Item:Row Number")
            n120 = Index Array(array=w229, index=w228) -> (element=w230:T26)
            n121 = Unbundle(w230) -> ("Operation"=w231:enum16{"Update", "Clear"}, "Color Box"=w232:u32)
            n122 = call <vilib>:"NT Read String.vi"("Name"="TestMode/TestName") -> ("String"=w226:string)  [unwired: 9 in, 1 out]
            n123 = call <vilib>:"NT Read and Format Entries as Tree.vi"("Operation"=w231, "Name Pattern"=w236, "Tree Refnum"=w237) -> ()  [unwired: 7 in, 2 out]
            n124 = case shown="\"\"" w226 {
              tunnel: "TestMode/TestProgress" ("Name") -> [w239 _]
              tunnel: "TestMode/TestProgressText" ("Name") -> [w238 _]
              frame Default {
                n125 = call <vilib>:"NT Read Number.vi"("Name"=w239) -> ("Numeric"=w240:dbl)  [unwired: 9 in, 1 out]
                n126 = call <vilib>:"NT Read String.vi"("Name"=w238) -> ("String"=w241:string)  [unwired: 9 in, 1 out]
                n127 = Bundle("Numeric"=w240, "String"=w241) -> (→"Progress":cluster{"Numeric":dbl, "String":string})  [unwired: 1 in]
              }
              frame "" {
                n128 = property on="Progress" class="Clust (strict)"("Visible"=FALSE) -> ()  [unwired: 2 in, 2 out]
                n129 = local write "Test Name"(u16 0) -> ()
              }
            }
            n130 = property on="Test Tree" class="Tree (strict)"("Active Item Row Number"=w235, "ActiveColNum"=w235, "CellBG"=w232, "Active Item Row Number"=-1 ("Active Item:Row Number"), "CellBG"=u32 5789784 ("Color Box")) -> ()  [unwired: 2 in, 2 out]
          }
          frame "Variables" {
            w247 = string[] ["CameraPublisher", "Usage", "DB"]  # Items to initially close
            n131 = First Call?() -> (First Call?: T/F=w248:bool)
            n132 = control-ref of="Tree"() -> (w249:refnum<vi>)
            n133 = Select(t=w247, s=w248, f=string[] []) -> (s? t:f=w245:string[])
            n134 = call <vilib>:"NT Read and Format Entries as Tree.vi"("Tags to  Close"=w245, "Tree Refnum"=w249) -> ()  [unwired: 8 in, 2 out]
          }
          frame "Commands" {
            w258 = u32 5789784 ("Color Box")
            w259 = T27 {"Row"=-1, "Column"=-2} ("Active Cell:Active Cell")
            w261 = T27 {"Row"=-2, "Column"=-2} ("Active Cell:Active Cell")
            n135 = Index Array(array=w262, index=w256) -> (element=w260:u32)
            n136 = Index Array(array=w257, index=w256) -> (element=w255:T26)
            n137 = Unbundle(w255) -> ("Operation"=w254:enum16{"Update", "Clear"})  [unwired: 1 out]
            n138 = local read "Command Selection"() -> (w253:i32)
            n139 = property on="Command Selection" class="MCListbox (strict)"("ActiveCell"=w261, "CellBG"=w260, "ActiveCell"=w259, "CellBG"=w258) -> ()  [unwired: 2 in, 2 out]
            n140 = call <vilib>:"WPI_DashboardUpdate RPC Info.vi"("Operation"=w254) -> ("update"=w252:bool, "commands"=w251:string[][])  [unwired: 9 in]
            n141 = property on="Command Selection" class="MCListbox (strict)"("ItemNames"=w251) -> ()  [unwired: 2 in, 2 out]
            n142 = property on="Command Params" class="Tbl (strict)"("Active Cell"=w261, "Cell BG Color"=w260, "Active Cell"=w259, "Cell BG Color"=w258) -> ()  [unwired: 2 in, 2 out]
            n143 = call <vilib>:"WPI_DashboardUpdate Command Params.vi"("Update"=w252, "NewVal"=w253, "Commands"=w251, "Param Tbl"=w250) -> ()  [unwired: 7 in, 1 out]
          }
        }
        n144 = call <vilib>:"Connextion Info.vi"() -> ("Connected"=→"NT Connection":bool)  [unwired: 10 in, 1 out]
      }
      event "Edit File": Value Change {
        n145 = event-data() -> ()  [unwired: 1 in, 6 out]
        n146 = property class="Ring (strict)"(reference=w274, error in=w273) -> (error out=w270:errorcluster, "Strings []"=w272:string[])  [unwired: 1 out]
        n147 = Index Array(array=w272, index="File") -> (element=w264:string)
        n148 = Build Path(base path=w263, name or relative path=w264) -> (appended path=w265:path)
        n149 = local write "Edit File"(FALSE ("Edit File")) -> ()
        n150 = call "Open File.vi"("error in (no error)"=w270, "appended path"=w265) -> ("error out"=w269:errorcluster)  [unwired: 9 in]
        n151 = call "Error Parser.vi"("error in (no error)"=w269) -> ("Explanation"=→"String":string, "error?"=→"Error":bool)  [unwired: 8 in, 1 out]
      }
      event "Click me if this is a new Driver Station": Value Change {
        n152 = event-data() -> ()  [unwired: 1 in, 6 out]
        n153 = local write "Click me if this is a new Driver Station"(FALSE ("Click me if this is a new Driver Station")) -> ()
        n154 = call "Create Symbolic Path to Public Documents.vi"() -> ()  [unwired: 12 in]
      }
      event "Transfer File": Value Change {
        n155 = event-data() -> ()  [unwired: 1 in, 6 out]
        n156 = property class="Ring (strict)"(reference=w291, error in=w281) -> (error out=w279:errorcluster, "Strings []"=w292:string[])  [unwired: 1 out]
        n157 = local read "File"() -> (w290:u16)
        n158 = Index Array(array=w292, index=w290) -> (element=w287:string)
        n159 = Build Path(base path=w288, name or relative path=w287) -> (appended path=w280:path)
        n160 = flat-sequence {
          tunnel: [w294] -> w278
          tunnel: w279 -> [w294]
          frame #0 {
            n161 = local write "String"("Sending file..." ("String")) -> ()
          }
        }
        n162 = call "Transfer file to roboRIO.vi"("error in (no error)"=w278, "Configuration File Path"=w280) -> ("error out"=w282:errorcluster, "String"=w283:string)  [unwired: 8 in]
        n163 = call "Error Parser.vi"("error in (no error)"=w282) -> ("Explanation"=w284:string, "error?"=w285:bool)  [unwired: 8 in, 1 out]
        n164 = Select(t=w284, s=w285, f=w283) -> (s? t:f=w286:string)
        n165 = local write "Transfer File"(FALSE ("Transfer File")) -> ()
        n166 = local write "Error"(w285) -> ()
        n167 = local write "String"(w286) -> ()
      }
      event "Retrieve File": Value Change {
        n168 = event-data() -> ()  [unwired: 1 in, 6 out]
        n169 = flat-sequence {
          tunnel: [w326] -> w300
          tunnel: w299 -> [w326]
          frame #0 {
            n170 = local write "String"("Retrieving file..." ("String")) -> ()
          }
        }
        n171 = property class="Ring (strict)"(reference=w313, error in=w300) -> (error out=w320:errorcluster, "Strings []"=w324:string[])  [unwired: 1 out]
        n172 = Format Date/Time String(time format string (%c)="%d%m%y%H%M%S.") -> (date/time string=w306:string)  [unwired: 2 in]
        n173 = call "Discover roboRIO.vi"("error in (no error)"=w320) -> ("error out"=w298:errorcluster, "roboRIO IP address"=w297:string)  [unwired: 8 in, 1 out]
        n174 = local read "File"() -> (w296:u16)
        n175 = Index Array(array=w324, index=w296) -> (element=w309:string)
        n176 = String To Path(string=w309) -> (path=w308:path)
        n177 = call <vilib>:"Get File Extension.vi"("file"=w308) -> ("unmodified file extension"=w307:string)  [unwired: 6 in, 4 out]
        n178 = Temporary Directory() -> (w310:path)
        n179 = Concatenate Strings(w306, w307) -> (w305:string)
        n180 = Concatenate Strings("/home/lvuser/" ("string"), w309) -> (w321:string)
        n181 = Build Path(base path=w310, name or relative path=w305) -> (appended path=w301:path)
        n182 = call <vilib>:"FTP Get File.vi"("password"="", "user"="Anonymous" ("username"), "error in (no error)"=w298, "local path"=w301, "remote path"=w321, "host"=w297) -> ("error out"=w319:errorcluster, "file error"=w318:errorcluster)  [unwired: 4 in]
        n183 = local write "Retrieve File"(FALSE ("Retrieve File")) -> ()
        n184 = Merge Errors(w318, w319) -> (w303:errorcluster)
        n185 = call "Open File.vi"("error in (no error)"=w303, "appended path"=w301) -> ("error out"=w302:errorcluster)  [unwired: 9 in]
        n186 = call "Error Parser.vi"("error in (no error)"=w302) -> ("Explanation"=w316:string, "error?"=w312:bool)  [unwired: 8 in, 1 out]
        n187 = Select(t=w316, s=w312, f="File read from the roboRIO successfully!") -> (s? t:f=w311:string)
        n188 = local write "Error"(w312) -> ()
        n189 = local write "String"(w311) -> ()
      }
      event "Open Personalities Tool": Value Change {
        w332 = refnum<vi> refnum ("type specifier VI Refnum (for type only)")
        n190 = event-data() -> ()  [unwired: 1 in, 6 out]
        n191 = feedback #1(w332) -> (w331:refnum<vi>)
        n192 = property class="VI Interface Type 0"(reference=w331) -> (reference out=w328:refnum<vi>, error out=w330:errorcluster, "FP.State"=w329:T23)  [unwired: 1 in]
        n193 = case shown="Default" w329 {
          tunnel: [w340 w344] -> w334
          tunnel: [w337 w343] -> w333
          tunnel: w332 -> [_ w352]
          tunnel: w328 -> [w341 w349]
          frame "Standard" {
            n194 = invoke class="VI (strict)" method="FP.Open"(reference=w341, "Activate"=TRUE ("Activate?"), "State"=T23."Standard") -> (reference out=w337:refnum<vi>, error out=w340:errorcluster)  [unwired: 2 in, 3 out]
          }
          frame Default {
            n195 = Close Reference(reference=w349) -> (error out=w350:errorcluster)  [unwired: 1 in]
            n196 = vi-ref "Personalities Tool.lvlib:Main.vi"() -> (w351:refnum<vi>)
            n197 = call <vilib>:"Clear Errors.vi"("error in (no error)"=w350) -> ("error out"=w347:errorcluster)  [unwired: 5 in, 1 out]
            n198 = property class="VI"(reference=w351, error in=w347) -> (error out=w348:errorcluster, "Path"=w353:path)  [unwired: 1 out]
            n199 = Open VI Reference(type specifier VI Refnum (for type only)=w352, vi path=w353, options=256, error in (no error)=w348) -> (vi reference=w345:refnum<vi>, error out=w346:errorcluster)  [unwired: 2 in]
            n200 = call-by-ref "Start Asynchronous Call"(reference=w345, error in=w346) -> (reference out=w343:refnum<vi>, error out=w344:errorcluster)  [unwired: 12 in]
          }
        }
        n201 = feedback-in #1(w333) -> ()
        n202 = call <vilib>:"Clear Errors.vi"("error in (no error)"=w330) -> ()  [unwired: 5 in, 2 out]
        n203 = local write "Open Personalities Tool"(FALSE ("Open Personalities Tool")) -> ()
        n204 = call <vilib>:"Simple Error Handler.vi"("error in (no error)"=w334) -> ()  [unwired: 4 in, 5 out]
      }
      event "Test Tree": Value Change {
        # "Show appropriate\ncontrols"
        n205 = event-data() -> ("CtlRef"=w358:refnum<vi>, "NewVal"=w356:string)  [unwired: 1 in]
        n206 = call <vilib>:"WPI_UtilitiesGetTreeIOName.vi"("NewVal"=w356, "TreeControl in"=w358) -> ("I/O Name"=w359:string)  [unwired: 9 in]
        n207 = case shown="\"Camera\"" w359 {
          selector: w359 -> [_ w366 _ w388 w397 _]
          tunnel: w356 -> [_ _ w385 w387 _ w404]
          tunnel: cluster{string[]}[] [{["640x480", "320x240", "160x120"]}, {["Auto", "Fixed indoor", "Fixed outdoor 1", "Fixed outdoor 2", "Fixed fluorescent 1", "Fixed fluorescent 2", "Hold current"]}, {["Auto", "Flicker-free 50 Hz", "Flicker-free 60 Hz", "Hold current"]}, {["None", "Prioritize frame rate", "Prioritize image quality"]}, {["Monochrome", "Color"]}] -> [_ _ _ _ _ w403]
          frame Default {
            w361 = FALSE ("Visible")
            w360 = FALSE ("Visible")
            n208 = property on="Motor" class="Clust (strict)"("Visible"=w360) -> ()  [unwired: 2 in, 2 out]
            n209 = property on="Test Ring" class="Ring (strict)"("Visible"=w360) -> ()  [unwired: 2 in, 2 out]
            n210 = property on="Rev/Fwd" class="Clust (strict)"("Visible"=w361) -> ()  [unwired: 2 in, 2 out]
            n211 = property on="On/Off" class="Bool (strict)"("Visible"=w361) -> ()  [unwired: 2 in, 2 out]
            n212 = property on="Test Slider" class="Slide (strict)"("Visible"=w361) -> ()  [unwired: 2 in, 2 out]
          }
          frame "Analog Out", "Motor", "PWM" {
            w367 = FALSE ("Visible")
            n213 = case shown="\"Analog Out\"" w366 {
              tunnel: [1.0 ("Value") -1.0 ("Value") 0.0 ("Value")] -> w365
              tunnel: [255.0 ("Value") 1.0 ("Value") 5.0 ("Value")] -> w364
              tunnel: [128.0 ("Value") 0.0 ("Value") 0.0 ("Value")] -> w363
              tunnel: [64.0 ("Value") 0.5 ("Value") 1.0 ("Value")] -> w362
              frame "PWM" {
              }
              frame "Motor", Default {
              }
              frame "Analog Out" {
              }
            }
            n214 = property on="Motor" class="Clust (strict)"("Visible"=TRUE) -> ()  [unwired: 2 in, 2 out]
            n215 = property on="Value" class="Slide (strict)"("Value"=w363, "Scale.Minimum"=w365, "Scale.Maximum"=w364, "Scale.Increment"=w362) -> ()  [unwired: 2 in, 2 out]
            n216 = property on="On/Off" class="Bool (strict)"("Visible"=w367) -> ()  [unwired: 2 in, 2 out]
            n217 = property on="Test Slider" class="Slide (strict)"("Visible"=w367) -> ()  [unwired: 2 in, 2 out]
            n218 = property on="Test Ring" class="Ring (strict)"("Visible"=w367) -> ()  [unwired: 2 in, 2 out]
            n219 = property on="Rev/Fwd" class="Clust (strict)"("Visible"=w367) -> ()  [unwired: 2 in, 2 out]
          }
          frame "Servo" {
            w383 = FALSE ("Visible")
            n220 = call <vilib>:"NT Read Number.vi"("Name"=w385) -> ("Numeric"=w384:dbl)  [unwired: 9 in, 1 out]
            n221 = property on="Test Slider" class="Slide (strict)"("Visible"=TRUE, "Scale.Maximum"=170.0 ("Scale.Range:Maximum")) -> ()  [unwired: 2 in, 2 out]
            n222 = local write "Test Slider"(w384) -> ()
            n223 = property on="Motor" class="Clust (strict)"("Visible"=w383) -> ()  [unwired: 2 in, 2 out]
            n224 = property on="Rev/Fwd" class="Clust (strict)"("Visible"=w383) -> ()  [unwired: 2 in, 2 out]
            n225 = property on="On/Off" class="Bool (strict)"("Visible"=w383) -> ()  [unwired: 2 in, 2 out]
            n226 = property on="Test Ring" class="Ring (strict)"("Visible"=w383) -> ()  [unwired: 2 in, 2 out]
          }
          frame "Relay", "Solenoid" {
            w386 = FALSE ("Visible")
            n227 = property on="Motor" class="Clust (strict)"("Visible"=w386) -> ()  [unwired: 2 in, 2 out]
            n228 = property on="Test Slider" class="Slide (strict)"("Visible"=w386) -> ()  [unwired: 2 in, 2 out]
            n229 = Search and Replace String(input string=w387, search string="/Value  **", replace string="/Direction") -> (result string=w393:string)  [unwired: 5 in, 3 out]
            n230 = property on="Test Ring" class="Ring (strict)"("Visible"=w386) -> ()  [unwired: 2 in, 2 out]
            n231 = call <vilib>:"NT Read String.vi"("Name"=w393) -> ("String"=w391:string)  [unwired: 9 in, 1 out]
            n232 = Equal?(x="Both directions", y=w391) -> (x = y?=w389:bool)
            n233 = Not(x=w389) -> (.not. x?=w390:bool)
            n234 = property on="Rev/Fwd" class="Clust (strict)"("Visible"=w389) -> ()  [unwired: 2 in, 2 out]
            n235 = property on="On/Off" class="Bool (strict)"("Visible"=w390, "Caption.Text"=w388) -> ()  [unwired: 2 in, 2 out]
          }
          frame "Compressor", "Digital Out" {
            w396 = FALSE ("Visible")
            # "Get direction and finish"
            n236 = property on="Motor" class="Clust (strict)"("Visible"=w396) -> ()  [unwired: 2 in, 2 out]
            n237 = property on="Test Slider" class="Slide (strict)"("Visible"=w396) -> ()  [unwired: 2 in, 2 out]
            n238 = property on="Test Ring" class="Ring (strict)"("Visible"=w396) -> ()  [unwired: 2 in, 2 out]
            n239 = property on="On/Off" class="Bool (strict)"("Visible"=TRUE, "Caption.Text"=w397) -> ()  [unwired: 2 in, 2 out]
            n240 = property on="Rev/Fwd" class="Clust (strict)"("Visible"=FALSE) -> ()  [unwired: 2 in, 2 out]
          }
          frame "Camera" {
            n241 = call <vilib>:"Get Last Path Segment.vi"("String in"=w404) -> ("String out"=w405:string)  [unwired: 10 in]
            n242 = property on="On/Off" class="Bool (strict)"("Visible"=FALSE) -> ()  [unwired: 2 in, 2 out]
            n243 = property on="Motor" class="Clust (strict)"("Visible"=FALSE) -> ()  [unwired: 2 in, 2 out]
            n244 = property on="Rev/Fwd" class="Clust (strict)"("Visible"=FALSE) -> ()  [unwired: 2 in, 2 out]
            n245 = case shown="\"White Balance  **\"" w405 {
              tunnel: w404 -> [w411 w420 w429 w438 w447 _ w453]
              tunnel: w403 -> [w409 w417 w426 w435 w444 _ _]
              frame "Size  **" {
                n246 = Index Array(array=w409) -> (element=w408:cluster{string[]})  [unwired: 1 in]
                n247 = call <vilib>:"NT Read String.vi"("Name"=w411) -> ("String"=w410:string)  [unwired: 9 in, 1 out]
                n248 = Unbundle(w408) -> (w406:string[])
                n249 = Match First String(2:w406, 3:w410) -> (0:w407:i32)  [unwired: 1 out]
                n250 = property on="Test Ring" class="Ring (strict)"("Value"=w407, "Strings []"=w406) -> ()  [unwired: 2 in, 2 out]
                n251 = property on="Test Ring" class="Ring (strict)"("Visible"=TRUE) -> ()  [unwired: 2 in, 2 out]
                n252 = property on="Test Slider" class="Slide (strict)"("Visible"=FALSE) -> ()  [unwired: 2 in, 2 out]
              }
              frame "White Balance  **" {
                n253 = Index Array(array=w417, index=1) -> (element=w418:cluster{string[]})
                n254 = call <vilib>:"NT Read String.vi"("Name"=w420) -> ("String"=w419:string)  [unwired: 9 in, 1 out]
                n255 = Unbundle(w418) -> (w415:string[])
                n256 = Match First String(2:w415, 3:w419) -> (0:w414:i32)  [unwired: 1 out]
                n257 = property on="Test Ring" class="Ring (strict)"("Value"=w414, "Strings []"=w415) -> ()  [unwired: 2 in, 2 out]
                n258 = property on="Test Ring" class="Ring (strict)"("Visible"=TRUE) -> ()  [unwired: 2 in, 2 out]
                n259 = property on="Test Slider" class="Slide (strict)"("Visible"=FALSE) -> ()  [unwired: 2 in, 2 out]
              }
              frame "Exposure  **" {
                n260 = Index Array(array=w426, index=2) -> (element=w427:cluster{string[]})
                n261 = call <vilib>:"NT Read String.vi"("Name"=w429) -> ("String"=w428:string)  [unwired: 9 in, 1 out]
                n262 = Unbundle(w427) -> (w423:string[])
                n263 = Match First String(2:w423, 3:w428) -> (0:w424:i32)  [unwired: 1 out]
                n264 = property on="Test Ring" class="Ring (strict)"("Value"=w424, "Strings []"=w423) -> ()  [unwired: 2 in, 2 out]
                n265 = property on="Test Ring" class="Ring (strict)"("Visible"=TRUE) -> ()  [unwired: 2 in, 2 out]
                n266 = property on="Test Slider" class="Slide (strict)"("Visible"=FALSE) -> ()  [unwired: 2 in, 2 out]
              }
              frame "Exposure Priority  **" {
                n267 = Index Array(array=w435, index=3) -> (element=w436:cluster{string[]})
                n268 = call <vilib>:"NT Read String.vi"("Name"=w438) -> ("String"=w437:string)  [unwired: 9 in, 1 out]
                n269 = Unbundle(w436) -> (w432:string[])
                n270 = Match First String(2:w432, 3:w437) -> (0:w433:i32)  [unwired: 1 out]
                n271 = property on="Test Ring" class="Ring (strict)"("Value"=w433, "Strings []"=w432) -> ()  [unwired: 2 in, 2 out]
                n272 = property on="Test Ring" class="Ring (strict)"("Visible"=TRUE) -> ()  [unwired: 2 in, 2 out]
                n273 = property on="Test Slider" class="Slide (strict)"("Visible"=FALSE) -> ()  [unwired: 2 in, 2 out]
              }
              frame "Color Enable  **" {
                n274 = Index Array(array=w444, index=4) -> (element=w445:cluster{string[]})
                n275 = call <vilib>:"NT Read String.vi"("Name"=w447) -> ("String"=w446:string)  [unwired: 9 in, 1 out]
                n276 = Unbundle(w445) -> (w441:string[])
                n277 = Match First String(2:w441, 3:w446) -> (0:w442:i32)  [unwired: 1 out]
                n278 = property on="Test Ring" class="Ring (strict)"("Value"=w442, "Strings []"=w441) -> ()  [unwired: 2 in, 2 out]
                n279 = property on="Test Ring" class="Ring (strict)"("Visible"=TRUE) -> ()  [unwired: 2 in, 2 out]
                n280 = property on="Test Slider" class="Slide (strict)"("Visible"=FALSE) -> ()  [unwired: 2 in, 2 out]
              }
              frame Default {
                n281 = property on="Test Ring" class="Ring (strict)"("Visible"=FALSE) -> ()  [unwired: 2 in, 2 out]
                n282 = property on="Test Slider" class="Slide (strict)"("Visible"=FALSE) -> ()  [unwired: 2 in, 2 out]
              }
              frame "Brightness  **", "Color Level  **", "Compression  **", "FPS  **", "Sharpness  **" {
                n283 = call <vilib>:"NT Read Number.vi"("Name"=w453) -> ("Numeric"=w452:dbl)  [unwired: 9 in, 1 out]
                n284 = local write "Test Slider"(w452) -> ()
                n285 = property on="Test Slider" class="Slide (strict)"("Visible"=TRUE, "Scale.Maximum"=100.0 ("Scale.Range:Maximum")) -> ()  [unwired: 2 in, 2 out]
                n286 = property on="Test Ring" class="Ring (strict)"("Visible"=FALSE) -> ()  [unwired: 2 in, 2 out]
              }
            }
          }
        }
        n287 = property on="Progress" class="Clust (strict)"("Visible"=FALSE) -> ()  [unwired: 2 in, 2 out]
      }
      event "Test Name": Mouse Enter {
        # "Populate the ring with the list of tests"
        n288 = event-data() -> ()  [unwired: 1 in, 1 out]
        n289 = call <vilib>:"NT Read String Array.vi"("Name"="TestMode/TestList") -> ("String Array"=w461:string[])  [unwired: 9 in, 1 out]
        n290 = Build Array (concatenate)("Select the test to run...", w461) -> (w460:string[])
        n291 = property on="Test Name" class="Ring (strict)"("Strings []"=w460) -> ()  [unwired: 2 in, 2 out]
      }
      event "Test Name": Value Change {
        w463 = FALSE ("Visible")
        # "Tell the robot the test name to run"
        n292 = event-data() -> ("NewVal"=w467:u16)  [unwired: 1 in]
        n293 = property on="Test Name" class="Ring (strict)"() -> ("Strings []"=w468:string[])  [unwired: 2 in, 2 out]
        n294 = local write "Progress"(T6 {"Test Progress"=0, "Test Progress Text"=""} ("Progress")) -> ()
        n295 = Index Array(array=w468, index=w467) -> (element=w466:string)
        n296 = call <vilib>:"NT Write String.vi"("String"=w466, "Name"="TestMode/TestName") -> ()  [unwired: 9 in, 1 out]
        n297 = property on="Progress" class="Clust (strict)"("Visible"=TRUE) -> ()  [unwired: 2 in, 2 out]
        n298 = property on="Motor" class="Clust (strict)"("Visible"=w463) -> ()  [unwired: 2 in, 2 out]
        n299 = property on="Test Slider" class="Slide (strict)"("Visible"=w463) -> ()  [unwired: 2 in, 2 out]
        n300 = property on="On/Off" class="Bool (strict)"("Visible"=w463) -> ()  [unwired: 2 in, 2 out]
        n301 = property on="Rev/Fwd" class="Clust (strict)"("Visible"=w463) -> ()  [unwired: 2 in, 2 out]
        n302 = property on="Test Ring" class="Ring (strict)"("Visible"=w463) -> ()  [unwired: 2 in, 2 out]
      }
      event "Select Auto": Mouse Enter {
        # "Populate the combo box with the list of autonomous options"
        n303 = event-data() -> ()  [unwired: 1 in, 1 out]
        n304 = call <vilib>:"NT Read String Array.vi"("Name"="Auto List") -> ("String Array"=w470:string[])  [unwired: 9 in, 1 out]
        n305 = property on="Select Auto" class="CmbBox"("Strings[]"=w470) -> ()  [unwired: 2 in, 2 out]
      }
      event "Select Auto": Value Change {
        # "User modified the Auto Selection. Write to NT variable so robot knows."
        n306 = event-data() -> ("NewVal"=w473:string)  [unwired: 1 in]
        n307 = call <vilib>:"NT Write String.vi"("String"=w473, "Name"="Auto Selector") -> ()  [unwired: 9 in, 1 out]
      }
      event "Command Selection": Value Change {
        # "Get the params and show in table"
        n308 = event-data() -> ("NewVal"=w479:i32)  [unwired: 1 in]
        n309 = property on="Command Selection" class="MCListbox (strict)"() -> ("ItemNames"=w477:string[][])  [unwired: 2 in, 2 out]
        n310 = call <vilib>:"WPI_DashboardUpdate Command Params.vi"("NewVal"=w479, "Commands"=w477, "Param Tbl"=w478) -> ()  [unwired: 8 in, 1 out]
      }
      event "Execute Command": Value Change {
        # "Started one, Unique ID holds\nresponse"
        n311 = event-data() -> ()  [unwired: 1 in, 1 out]
        n312 = property on="Command Selection" class="MCListbox (strict)"() -> ("ItemNames"=w490:string[][])  [unwired: 2 in, 2 out]
        n313 = Index Array(array=w490, index (row)="Command Selection", index (col)=0) -> (element=w488:string)
        n314 = call <vilib>:"Invoke Commands.vi"("Command Params"="Command Params", "Function Name"=w488) -> ("Params"=w484:u8, "Started"=w483:bool)  [unwired: 7 in, 1 out]
        n315 = Array Subset(array="Command Params", length (row)=w484) -> (w485:string[][])  [unwired: 3 in]
        n316 = Select(t="Executing" ("Cmd Status"), s=w483, f="" ("Cmd Status")) -> (s? t:f=→"Cmd Status":string)
      }
      event "Command Selection": Double Click {
        n317 = event-data() -> ("Row"=w498:i32)  [unwired: 1 in]
        n318 = property on="Command Selection" class="MCListbox (strict)"() -> ("ItemNames"=w501:string[][])  [unwired: 2 in, 2 out]
        n319 = local read "Command Params"() -> (w497:string[][])
        n320 = Index Array(array=w501, index (row)=w498, index (col)=0) -> (element=w499:string)
        n321 = call <vilib>:"Invoke Commands.vi"("Command Params"=w497, "Function Name"=w499) -> ("Params"=w496:u8, "Started"=w491:bool)  [unwired: 7 in, 1 out]
        n322 = Array Subset(array=w497, length (row)=w496) -> (w495:string[][])  [unwired: 3 in]
        n323 = Select(t="Executing" ("Cmd Status"), s=w491, f="" ("Cmd Status")) -> (s? t:f=w492:string)
        n324 = local write "Cmd Status"(w492) -> ()
      }
      event "CheckList": Double Click {
        # "Shift clears all"
        # "Update symbols on the listbox"
        n325 = event-data() -> ("PlatMods.Shift"=w503:bool, "Row"=w505:i32)  [unwired: 1 in]
        n326 = case shown="True" w503 {
          tunnel: w505 -> [w509 _]
          tunnel: 1 -> [w508 _]
          frame False {
            n327 = property on="CheckList" class="LstBox (strict)"() -> ("Item Symbols"=w507:i32[])  [unwired: 2 in, 2 out]
            n328 = Replace Array Subset(array=w507, new element=w508, index=w509) -> (w506:i32[])
            n329 = property on="CheckList" class="LstBox (strict)"("Item Symbols"=w506) -> ()  [unwired: 2 in, 2 out]
          }
          frame True {
            w510 = 0 ("Top Row")
            n330 = property on="CheckList" class="LstBox (strict)"() -> ("Number of Rows"=w512:u32)  [unwired: 2 in, 2 out]
            n331 = Initialize Array(0, w512) -> (w511:i32[])
            n332 = property on="CheckList" class="LstBox (strict)"("Top Row"=w510, "Value"=w510, "Item Symbols"=w511) -> ()  [unwired: 2 in, 2 out]
          }
        }
      }
      event "CheckList": Key Down {
        # "Update symbols on the listbox\nLeft and right keys check and uncheck"
        n333 = event-data() -> ("VKey"=w516:T24)  [unwired: 1 in]
        n334 = case shown="\"Left\", \"Right\"" w516 {
          selector: w516 -> [w521 _]
          tunnel: eventvkey."Left" ("VKey") -> [w519 _]
          frame "Left", "Right" {
            n335 = Equal?(x=w519, y=w521) -> (x = y?=w520:bool)
            n336 = Select(t=0, s=w520, f=1) -> (s? t:f=w522:i32)
            n337 = property on="CheckList" class="LstBox (strict)"() -> ("Item Symbols"=w525:i32[])  [unwired: 2 in, 2 out]
            n338 = Replace Array Subset(array=w525, new element=w522, index="CheckList") -> (w524:i32[])
            n339 = property on="CheckList" class="LstBox (strict)"("Item Symbols"=w524) -> ()  [unwired: 2 in, 2 out]
          }
          frame Default {
          }
        }
      }
      event "Motor.Enable": Value Change {
        # "When the test mode otor enable helper is set, update that\ntree row item's value"
        n340 = event-data() -> ("NewVal"=w531:bool)  [unwired: 1 in]
        n341 = Unbundle("Motor") -> ("Value"=w530:dbl)  [unwired: 1 out]
        n342 = Select(t=w530, s=w531, f=0.0) -> (s? t:f=w528:dbl)
        n343 = call <vilib>:"NT Write Number.vi"("Numeric"=w528, "Name"=w527) -> ()  [unwired: 9 in, 1 out]
      }
      event "Test Slider": Value Change {
        # "When the test mode slider helper is set, update that\ntree row item's value"
        n344 = event-data() -> ("NewVal"=w534:dbl)  [unwired: 1 in]
        n345 = call <vilib>:"NT Write Number.vi"("Numeric"=w534, "Name"=w535) -> ()  [unwired: 9 in, 1 out]
      }
      event "On/Off": Value Change {
        # "When the test mode on/off helper value is set, update that\ntree row item's value"
        n346 = event-data() -> ("NewVal"=w539:bool)  [unwired: 1 in]
        n347 = Boolean To (0,1)(Boolean=w539) -> (0, 1=w538:i16)
        n348 = call <vilib>:"NT Write Number.vi"("Numeric"=w538, "Name"=w537) -> ()  [unwired: 9 in, 1 out]
      }
      event "Rev/Fwd": Value Change {
        # "When the test mode helper value for relays is set, update that\ntree row item's value"
        n349 = event-data() -> ("NewVal.Forward"=w547:bool, "NewVal.Reverse"=w546:bool)  [unwired: 1 in]
        n350 = Boolean To (0,1)(Boolean=w547) -> (0, 1=w543:i16)
        n351 = Boolean To (0,1)(Boolean=w546) -> (0, 1=w545:i16)
        n352 = Negate(x=w545) -> (-x=w544:i16)
        n353 = Add(x=w543, y=w544) -> (x+y=w542:i16)
        n354 = call <vilib>:"NT Write Number.vi"("Numeric"=w542, "Name"=w541) -> ()  [unwired: 9 in, 1 out]
      }
      event "Test Ring": Value Change {
        # "When a test mode helper value is selected from the ring,\nset the tree item's variable to the string value"
        n355 = event-data() -> ("NewVal"=w551:u16)  [unwired: 1 in]
        n356 = property on="Test Ring" class="Ring (strict)"() -> ("Strings []"=w552:string[])  [unwired: 2 in, 2 out]
        n357 = Index Array(array=w552, index=w551) -> (element=w550:string)
        n358 = call <vilib>:"NT Write String.vi"("String"=w550, "Name"=w549) -> ()  [unwired: 9 in, 1 out]
      }
      event "Rec Mode": Value Change {
        # "Update globals for recording mode and path to read log from.\nClear when logging and let NetworkTables set path for vision to\nuse."
        n359 = event-data() -> ("NewVal"=w563:enum32{"Stop", "Record", "Playback"})  [unwired: 1 in]
        n360 = global write "WPI_DashboardLogging Global.vi" "Logging Filename"(path "") -> ()
        n361 = global write "WPI_DashboardLogging Global.vi" "Recording"(w563) -> ()
        n362 = case shown="\"Playback\"" w563 {
          tunnel: w562 -> [_ w565 w574]
          tunnel: [_ _ w573] -> w560
          tunnel: [_ _ w572] -> _
          tunnel: w558 -> [_ _ w570]
          tunnel: cluster{i32, i32} {-250, 170} -> [_ _ w569]
          tunnel: [_ _ T25 {"Image Size"=TRUE, "Image Type"=TRUE, "Pixel Value"=TRUE, "ROI Information"=TRUE, "Zoom Factor"=FALSE} ("Image Information Shown:All Elements")] -> w553
          tunnel: [_ _ TRUE ("Zoom Factor")] -> w554
          tunnel: w556 -> [_ _ w566]
          frame Default {
          }
          frame "Stop", "Record" {
            # "Place Window too"
            n363 = invoke class="VI" method="FP.Close"(reference=w565) -> (reference out=w564:refnum<vi>)  [unwired: 2 in, 2 out]
            n364 = invoke class="VI" method="Abort VI"(reference=w564) -> ()  [unwired: 2 in, 3 out]
          }
          frame "Playback" {
            n365 = call "Open Playback Panel.vi"("Offset"=w569, "DB VI Ref"=w570, "Playback in"=w574) -> ("Playback out"=w571:refnum<vi>)  [unwired: 8 in]
            n366 = register-events(w571, w566) -> (reference out=w573:refnum<event-registration>, error out=w572:errorcluster)  [unwired: 2 in]
          }
        }
        n367 = property on="Camera Image Right" class="ImageControl"("Image Information Shown"=w553, "Image Information Visible"=w554) -> ()  [unwired: 2 in, 2 out]
        n368 = property on="Camera Image" class="ImageControl"("Image Information Shown"=w553, "Image Information Visible"=w554) -> ()  [unwired: 2 in, 2 out]
        n369 = call <vilib>:"WPI_DashboardNT Log FieldName Cache.vi"("Operation"=enum16{"Lookup/Add", "Index", "Clear"}."Clear") -> ()  [unwired: 8 in, 3 out]
      }
      event Panel Close {
        w576 = enum32{"Stop", "Record", "Playback"}."Stop" ("Rec Mode")
        # "Playback window has been closed, abort"
        n370 = event-data() -> ()  [unwired: 1 in, 4 out]
        n371 = local write "Rec Mode"(w576) -> ()
        n372 = global write "WPI_DashboardLogging Global.vi" "Recording"(w576) -> ()
      }
      event Panel Close {
        # "Abort playback window and ourself"
        n373 = event-data() -> ()  [unwired: 1 in, 4 out]
        n374 = invoke class="VI" method="FP.Close"(reference=w580) -> (reference out=w579:refnum<vi>)  [unwired: 2 in, 2 out]
        n375 = invoke class="VI" method="Abort VI"(reference=w579) -> (error out=w578:errorcluster)  [unwired: 2 in, 2 out]
        n376 = invoke class="VI" method="Abort VI"(error in=w578) -> ()  [unwired: 2 in, 3 out]
      }
      event User Event {
        n377 = event-data() -> ("IDs"=w587:cluster{"RPC field ID":u16, "Unique ID":u16}, "String"=w586:string)  [unwired: 1 in]
        n378 = Bundle("IDs"=w587, "String"=w586) -> (w585:T10)  [unwired: 1 in]
        n379 = call <vilib>:"Retrieve RPC Response.vi"("RPC Response"=w585) -> ("Output"=w583:string[][])  [unwired: 10 in]
        n380 = Build Array (concatenate)(w581, w583) -> (w582:string[][])
        n381 = local write "Command Params"(w582) -> ()
        n382 = local write "Cmd Status"("" ("Cmd Status")) -> ()
      }
      event "Tree": Double Click {
        n383 = event-data() -> ("PlatMods"=w593:T28, "Tag"=w590:string)  [unwired: 1 in]
        n384 = Unbundle(w593) -> ("Shift"=w592:bool)  [unwired: 4 out]
        n385 = String Subset(string=w590, length (rest)=1 ("length (rest)")) -> (substring=w589:string)  [unwired: 1 in]
        n386 = Not(x=w592) -> (.not. x?=w591:bool)
        n387 = case shown="\"/\"" w589 {
          tunnel: w590 -> [_ w596]
          tunnel: w591 -> [_ w595]
          frame Default {
          }
          frame "/" {
            n388 = call <vilib>:"NT Update Persistence.vi"("Persistence"=w595, "Name"=w596) -> ()  [unwired: 9 in, 1 out]
          }
        }
      }
    }
  }
  n389 = while {
    tunnel: w76 -> [w598]
    i -> [w601]
    stop <- FALSE stop-if-true
    n390 = Wait (ms)(milliseconds to wait=u32 100) -> ()  [unwired: 1 out]
    n391 = case shown="\"Playback\"" "Rec Mode" {
      tunnel: w601 -> [_ _ w616]
      tunnel: [u32 2829099 ("Base Color") u32 11141120 ("Target Color") w605] -> w597
      frame "Stop", Default {
        # "Reset the color, extra updates don't cost much"
      }
      frame "Record" {
      }
      frame "Playback" {
        # "Playback"
        n392 = Quotient & Remainder(x=w616, y=u32 50 ("milliseconds to wait")) -> (x-y*floor(x/y)=w612:u32)  [unwired: 1 out]
        n393 = Divide(x=w612, y=u32 50 ("milliseconds to wait")) -> (x/y=w609:dbl)
        n394 = Multiply(x=6.283185307179586, y=w609) -> (x*y=w614:dbl)
        n395 = Sine(x=w614) -> (sin(x)=w613:dbl)
        n396 = Absolute Value(x=w613) -> (abs(x)=w606:dbl)
        n397 = call "Interpolate RGB Color.vi"("Proportion"=w606, "Target Color"=u32 30976, "Base Color"=u32 2829099) -> ("Result Color"=w605:u32)  [unwired: 8 in]
      }
    }
    n398 = property class="Pane"(reference=w598, "PaneColor"=w597) -> ()  [unwired: 1 in, 2 out]
  }
  n399 = local write "Dashboard Tab"(T2."Drive" ("Dashboard Tab")) -> ()
  n400 = property on="On/Off" class="Bool (strict)"("Visible"=w47) -> ()  [unwired: 2 in, 2 out]
  n401 = property on="Motor" class="Clust (strict)"("Visible"=w47) -> ()  [unwired: 2 in, 2 out]
  n402 = property on="Progress" class="Clust (strict)"("Visible"=w47) -> ()  [unwired: 2 in, 2 out]
  n403 = property on="Test Ring" class="Ring (strict)"("Visible"=w47) -> ()  [unwired: 2 in, 2 out]
  n404 = property on="Rev/Fwd" class="Clust (strict)"("Visible"=w47) -> ()  [unwired: 2 in, 2 out]
  n405 = while {
    tunnel: u16 1741 ("timeout ms (25000)") -> [w618]
    stop <- FALSE stop-if-true
    n406 = TCP Create Listener(10:w618) -> (0:w617:errorcluster, 3:w619:refnum<k5>)  [unwired: 4 in, 1 out]
    n407 = case shown="No Error" w617 {
      selector: w617 -> [w621 _]
      tunnel: w619 -> [w622 _]
      frame No Error {
        n408 = while {
          tunnel: w622 -> [w625]
          tunnel: w621 -> [w624]
          stop <- FALSE stop-if-true
          n409 = TCP Wait On Listener(8:w624, 11:w625) -> (0:w626:errorcluster, 4:w627:refnum<k5>)  [unwired: 2 in, 3 out]
          n410 = local write "TCP"(w627) -> ()
          n411 = case shown="No Error" w626 {
            frame No Error {
            }
            frame Error {
              n412 = Wait (ms)(milliseconds to wait=u32 1000) -> ()  [unwired: 1 out]
            }
          }
        }
      }
      frame Error {
        n413 = Wait (ms)(milliseconds to wait=u32 1000) -> ()  [unwired: 1 out]
      }
    }
  }
  n414 = local write "Command Selection"(u16 0 ("milliseconds to wait")) -> ()
  n415 = local write "Command Params"(string[][] [] ("Command Params")) -> ()
  n416 = global write "WPI_DashboardLogging Global.vi" "Recording"(w70) -> ()
  n417 = local write "Rec Mode"(w70) -> ()
  n418 = call <vilib>:"NT Write String.vi"("String"="Select Auto", "Name"="Auto Selector") -> ()  [unwired: 9 in, 1 out]
